vi "MouseMoveAllY.vi"(8 "YNum":i32, 10 "Delta":i32, 11 "XYGraph输入":refnum<vi>) -> ()   [LabVIEW 2015]
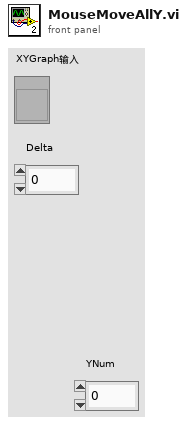
[diagram p1: front panel]
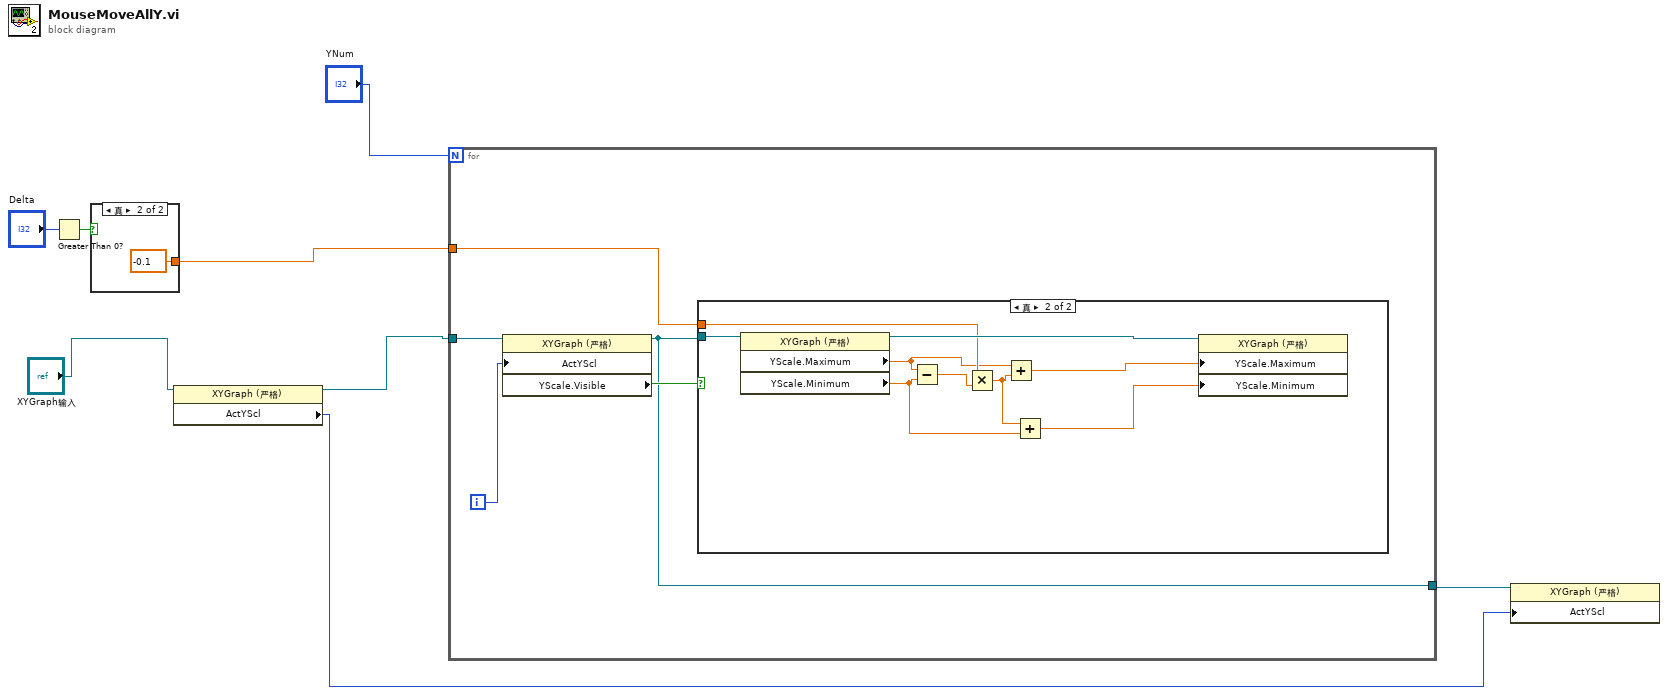
[diagram p0: block diagram]
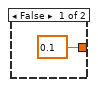
[diagram p3: hidden frame]
diagram:
  n1 = Greater Than 0?(x="Delta") -> (x > 0?=w8:bool)
  n2 = case shown="真" w8 {
    tunnel: [0.1 -0.1] -> w6
    frame False {
    }
    frame True {
    }
  }
  n3 = property class="XYGraph (严格)"(reference="XYGraph输入") -> (reference out=w3:refnum<vi>, "ActYScl"=w1:i32)  [unwired: 1 in, 1 out]
  n4 = for {
    N: "YNum" -> [_]
    tunnel: w3 -> [w13]
    tunnel: w6 -> [w15]
    tunnel: [w11] -> w2
    i -> [w12]
    n5 = property class="XYGraph (严格)"(reference=w13, "ActYScl"=w12) -> (reference out=w11:refnum<vi>, "YScale.Visible"=w14:bool)  [unwired: 1 in, 1 out]
    n6 = case shown="真" w14 {
      tunnel: w11 -> [_ w23]
      tunnel: w15 -> [_ w21]
      frame False {
      }
      frame True {
        n7 = property class="XYGraph (严格)"(reference=w23) -> (reference out=w24:refnum<vi>, "YScale.Maximum"=w20:dbl, "YScale.Minimum"=w18:dbl)  [unwired: 1 in, 1 out]
        n8 = Subtract(x=w20, y=w18) -> (x-y=w22:dbl)
        n9 = Multiply(x=w21, y=w22) -> (x*y=w19:dbl)
        n10 = Add(x=w20, y=w19) -> (x+y=w17:dbl)
        n11 = Add(x=w19, y=w18) -> (x+y=w16:dbl)
        n12 = property class="XYGraph (严格)"(reference=w24, "YScale.Maximum"=w17, "YScale.Minimum"=w16) -> ()  [unwired: 1 in, 2 out]
      }
    }
  }
  n13 = property class="XYGraph (严格)"(reference=w2, "ActYScl"=w1) -> ()  [unwired: 1 in, 2 out]
